vi "myFFT.vi"(11 "Array in":dbl[](array[numeric])) -> (2 "Array out":dbl[](array[numeric]), 3 "FFT {X}":cdb[](array[numeric]))   [LabVIEW 2018]
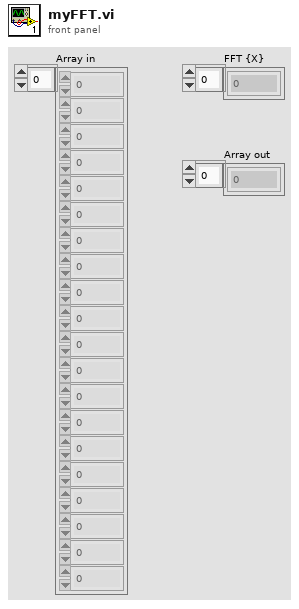
[diagram p1: front panel]
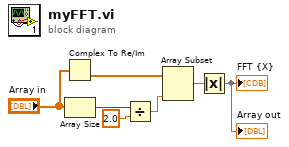
[diagram p0: block diagram]
diagram:
  n1 = Complex To Re/Im(x + iy="Array in") -> (y=w3:dbl[])  [unwired: 1 out]
  n2 = Array Size(array="Array in") -> (size(s)=w5:i32)
  n3 = Divide(x=w5, y=2.0) -> (x/y=w6:dbl)
  n4 = Array Subset(array=w3, length=w6) -> (w7:dbl[])  [unwired: 1 in]
  n5 = Absolute Value(x=w7) -> (abs(x)=→"Array out" →"FFT {X}":dbl[])
